vi "Drive Mode Cleaned.vi"   [LabVIEW 2018]
types:
  T1 = enum16{"Name Contains", "Name Equals", "HID Type", "XBox Type", "Axis Count", "Axis Type", "Button Count", "POV Count"}[]
  T2 = typedef "WPI_JoystickDeviceEnum.ctl" = enum16{"USB 0", "USB 1", "USB 2", "USB 3", "USB 4", "USB 5"}
  T3 = cluster{"[0]":bool, "[1]":bool, "[2]":bool, "[3]":bool, "[4]":bool, "[5]":bool, "[6]":bool, "[7]":bool, "[8]":bool}
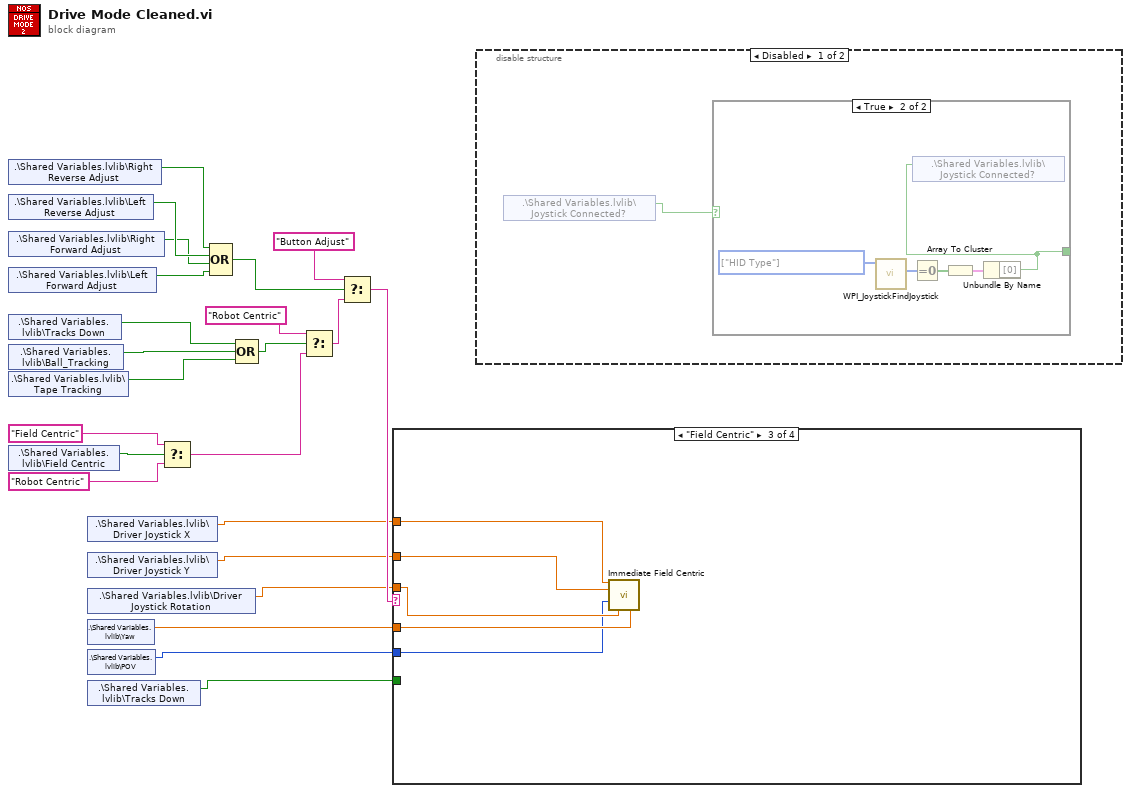
[diagram p0: block diagram]
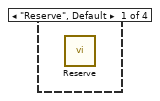
[diagram p4: hidden frame]
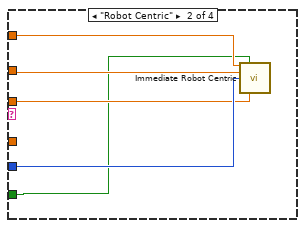
[diagram p5: hidden frame]
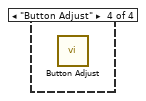
[diagram p6: hidden frame]
diagram:
  n1 = shared-variable ".\\Shared Variables.lvlib\\Right Reverse Adjust"() -> (w9:bool)  [unwired: 1 in, 1 out]
  n2 = shared-variable ".\\Shared Variables.lvlib\\Left Reverse Adjust"() -> (w8:bool)  [unwired: 1 in, 1 out]
  n3 = shared-variable ".\\Shared Variables.lvlib\\Right Forward Adjust"() -> (w7:bool)  [unwired: 1 in, 1 out]
  n4 = shared-variable ".\\Shared Variables.lvlib\\Left Forward Adjust"() -> (w6:bool)  [unwired: 1 in, 1 out]
  n5 = shared-variable ".\\Shared Variables.lvlib\\Tracks Down"() -> (w4:bool)  [unwired: 1 in, 1 out]
  n6 = shared-variable ".\\Shared Variables.lvlib\\Ball_Tracking"() -> (w3:bool)  [unwired: 1 in, 1 out]
  n7 = shared-variable ".\\Shared Variables.lvlib\\Tape Tracking"() -> (w2:bool)  [unwired: 1 in, 1 out]
  n8 = shared-variable ".\\Shared Variables.lvlib\\Field Centric"() -> (w22:bool)  [unwired: 1 in, 1 out]
  n9 = shared-variable ".\\Shared Variables.lvlib\\Driver Joystick X"() -> (w18:dbl)  [unwired: 1 in, 1 out]
  n10 = shared-variable ".\\Shared Variables.lvlib\\Driver Joystick Y"() -> (w17:dbl)  [unwired: 1 in, 1 out]
  n11 = shared-variable ".\\Shared Variables.lvlib\\Driver Joystick Rotation"() -> (w16:dbl)  [unwired: 1 in, 1 out]
  n12 = shared-variable ".\\Shared Variables.lvlib\\Yaw"() -> (w15:dbl)  [unwired: 1 in, 1 out]
  n13 = shared-variable ".\\Shared Variables.lvlib\\POV"() -> (w14:i16)  [unwired: 1 in, 1 out]
  n14 = shared-variable ".\\Shared Variables.lvlib\\Tracks Down"() -> (w13:bool)  [unwired: 1 in, 1 out]
  n15 = Select(t="Field Centric", s=w22, f="Robot Centric") -> (s? t:f=w11:string)
  n16 = Compound Arithmetic op=OR(w9, w8, w7, w6) -> (w5:bool)
  n17 = Compound Arithmetic op=OR(w4, w3, w2) -> (w1:bool)
  n18 = Select(t="Robot Centric", s=w1, f=w11) -> (s? t:f=w12:string)
  n19 = Select(t="Button Adjust", s=w5, f=w12) -> (s? t:f=w19:string)
  n20 = case shown="\"Field Centric\"" w19 {
    tunnel: w18 -> [_ w28 w33 _]
    tunnel: w17 -> [_ w27 w32 _]
    tunnel: w16 -> [_ w25 w30 _]
    tunnel: w15 -> [_ _ w31 _]
    tunnel: w14 -> [_ w26 w29 _]
    tunnel: w13 -> [_ w24 _ _]
    frame "Reserve", Default {
      n21 = call "Reserve.vi"() -> ()  [unwired: 11 in, 1 out]
    }
    frame "Robot Centric" {
      n22 = call "Immediate Robot Centric.vi"("X Setpoint"=w28, "Tracks"=w24, "Y Setpoint"=w27, "POV"=w26, "Z Setpoint"=w25) -> ()  [unwired: 10 in, 1 out]
    }
    frame "Field Centric" {
      n23 = call "Immediate Field Centric.vi"("X Setpoint"=w33, "Y Setpoint"=w32, "POV"=w29, "Z Setpoint"=w30, "Gyro"=w31) -> ()  [unwired: 10 in, 1 out]
    }
    frame "Button Adjust" {
      n24 = call "Button Adjust.vi"() -> ()  [unwired: 11 in, 1 out]
    }
  }
  n25 = disable-structure shown="Disabled" {
    frame Disabled {
      n26 = shared-variable ".\\Shared Variables.lvlib\\Joystick Connected?"() -> (w34:bool)  [unwired: 1 in, 1 out]
      n27 = case shown="True" w34 {
        selector: w34 -> [w35 _]
        tunnel: [w35 w36] -> _
        frame False {
        }
        frame True {
          w40 = T1 [enum."HID Type"] items=["Name Contains", "Name Equals", "HID Type", "XBox Type", "Axis Count", "Axis Type", "Button Count", "POV Count"] ("Match Criteria")
          n28 = call <vilib>:"WPI_JoystickFindJoystick.vi"("Match Criteria"=w40) -> ("Matching Joysticks"=w39:T2[])  [unwired: 9 in, 1 out]
          n29 = Equal To 0?(x=w39) -> (x = 0?=w38:bool[])
          n30 = Array To Cluster(array=w38) -> (cluster=w37:T3)
          n31 = Unbundle By Name(w37) -> ("[0]"=w36:bool)
          n32 = shared-variable ".\\Shared Variables.lvlib\\Joystick Connected?"(w36) -> ()  [unwired: 1 in, 1 out]
        }
      }
    }
    frame Enabled {
    }
  }
